vi "GetRowColumn.vi"(8 "error":errorcluster caption="错误输入（无错误）", 11 "Excel._Worksheet":refnum<k7>) -> (0 "error out":errorcluster caption="错误输出", 1 "CountColumn":i32, 2 "CountRow":i32, 3 "Excel._Worksheet":refnum<k7>)   [LabVIEW 2017]
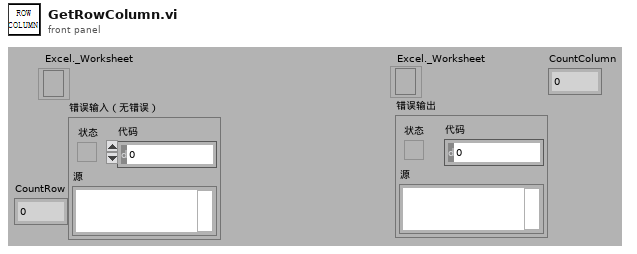
[diagram p1: front panel]
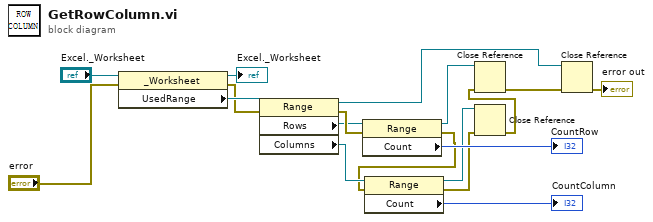
[diagram p0: block diagram]
diagram:
  n1 = property class="_Worksheet"(reference="Excel._Worksheet", error in="error") -> (reference out=→"Excel._Worksheet":refnum<k7>, error out=w16:errorcluster, "UsedRange"=w18:refnum<k7>)
  n2 = property class="Range"(reference=w18, error in=w16) -> (reference out=w11:refnum<k7>, error out=w15:errorcluster, "Rows"=w8:refnum<k7>, "Columns"=w3:refnum<k7>)
  n3 = property class="Range"(reference=w8, error in=w15) -> (reference out=w6:refnum<k7>, error out=w2:errorcluster, "Count"=→"CountRow":i32)
  n4 = property class="Range"(reference=w3, error in=w2) -> (reference out=w5:refnum<k7>, error out=w4:errorcluster, "Count"=→"CountColumn":i32)
  n5 = Close Reference(reference=w5, error in (no error)=w4) -> (error out=w1:errorcluster)
  n6 = Close Reference(reference=w6, error in (no error)=w1) -> (error out=w14:errorcluster)
  n7 = Close Reference(reference=w11, error in (no error)=w14) -> (error out=→"error out":errorcluster)
